vi "MiniCanSat 2018 V1.1.vi"() -> ()   [LabVIEW 2015]
uses:
  <vilib>/Instr/_visa.llb/VISA Configure Serial Port (Instr).vi
panel:
  out "Waveform Chart":dbl(graph)=145.63
  out "XY Graph":cluster{dbl[], dbl[]}(graph)={[100.91229833333334, 100.91229833333334, 100.91229999999999, 100.91229833333334, 100.912295, 100.912295, 100.912295, 100.912295, 100.912295, 100.91229666666668, 100.91229833333334, 100.91229833333334, 100.91229666666668, 100.91229833333334, 100.91229833333334, 100.91229999999999, 100.91229999999999, 100.91230166666668, 100.91230166666668, 100.91229999999999, 100.91229833333334, 100.912295, 100.91229333333334, 100.91229666666668, 100.91229666666668, 100.912295, 100.91229166666666, 100.91228833333335, 100.91228666666666, 100.91228500000001, 100.91228166666666, 100.91227833333332, 100.91227833333332, 100.91227666666667, 100.91227666666667, 100.91227500000001, 100.91227500000001, 100.91227333333333, 100.91227333333333, 100.91227333333333, 100.91227333333333, 100.91227333333333, 100.91227333333333, 100.91227333333333, 100.91227500000001, 100.91227500000001, 100.91227666666667, 100.91228166666666, 100.91228500000001, 100.91228833333335, 100.91229, 100.91229166666666, 100.91229166666666, 100.912295, 100.91229666666668, 100.91229999999999, 100.91230166666668, 100.91230166666668, 100.91229999999999, 100.91229833333334, 100.912295, 100.91229166666666, 100.91228666666666, 100.91228833333335, 100.91228666666666, 100.91228500000001, 100.91228166666666, 100.91227500000001, 100.91227500000001, 100.91227333333333, 100.91227666666667, 100.91227500000001, 100.91227333333333, 100.91227833333332, 100.91227500000001, 100.91227500000001, 100.91227833333332, 100.91228333333332, 100.91228666666666, 100.91229166666666, 100.912295, 100.91229833333334, 100.91230166666668, 100.91230333333333, 100.91230500000002, 100.91230666666667, 100.91230833333333, 100.91230833333333, 100.91231, 100.91231, 100.91231333333332, 100.912315, 100.91231333333332, 100.912315, 100.91231333333332, 100.91231333333332, 100.91231666666665, 100.91232166666666, 100.91232, 100.91232166666666, 100.91232166666666, 100.91232333333333, 100.91232333333333, 100.91232333333333, 100.91232666666669, 100.91233333333334, 100.91233333333334, 100.91233500000001, 100.91233666666668, 100.91233666666668, 100.91233500000001, 100.91233833333332, 100.91234166666666, 100.91234000000001, 100.91233833333332, 100.91234000000001, 100.91234166666666, 100.91234333333333, 100.91234333333333, 100.91234666666666, 100.91235, 100.91235166666665, 100.91235333333334, 100.91235333333334, 100.91235, 100.91234666666666, 100.912345, 100.91234000000001, 100.91233500000001, 100.91233333333334, 100.91233500000001, 100.91233333333334, 100.91233166666667, 100.91232999999998, 100.91232833333333, 100.91232666666669, 100.91233500000001, 100.91233166666667], [15.036158333333333, 15.036156666666667, 15.036156666666667, 15.036155, 15.036153333333335, 15.036155, 15.036155, 15.036155, 15.036155, 15.036155, 15.036155, 15.036155, 15.036153333333335, 15.036153333333335, 15.036153333333335, 15.036153333333335, 15.036153333333335, 15.036155, 15.036156666666667, 15.036158333333333, 15.036161666666665, 15.036161666666665, 15.03616333333333, 15.036166666666668, 15.036168333333334, 15.03617, 15.036173333333332, 15.036178333333332, 15.036181666666668, 15.036183333333334, 15.036183333333334, 15.036185, 15.036185, 15.036185, 15.036185, 15.036183333333334, 15.036183333333334, 15.036183333333334, 15.036181666666668, 15.036181666666668, 15.036180000000002, 15.036176666666666, 15.036174999999998, 15.036174999999998, 15.036176666666666, 15.036176666666666, 15.036178333333332, 15.036178333333332, 15.036178333333332, 15.036176666666666, 15.036174999999998, 15.036173333333332, 15.036171666666666, 15.03617, 15.036168333333334, 15.036166666666668, 15.036161666666665, 15.036156666666667, 15.036155, 15.036153333333335, 15.036153333333335, 15.036153333333335, 15.036151666666667, 15.036151666666667, 15.036153333333335, 15.036153333333335, 15.036155, 15.036156666666667, 15.036159999999999, 15.036159999999999, 15.03616333333333, 15.036165000000002, 15.036166666666668, 15.03617, 15.03617, 15.036171666666666, 15.036176666666666, 15.036181666666668, 15.036185, 15.036188333333333, 15.03619, 15.036193333333332, 15.036196666666667, 15.036198333333335, 15.036200000000001, 15.036203333333333, 15.036203333333333, 15.036204999999999, 15.036204999999999, 15.036204999999999, 15.036204999999999, 15.036203333333333, 15.036201666666667, 15.036201666666667, 15.036203333333333, 15.036204999999999, 15.036206666666665, 15.036210000000002, 15.036213333333334, 15.036218333333332, 15.036221666666666, 15.036221666666666, 15.036223333333332, 15.036223333333332, 15.036223333333332, 15.036223333333332, 15.036221666666666, 15.036219999999998, 15.036218333333332, 15.036216666666666, 15.036215, 15.036211666666668, 15.036210000000002, 15.036210000000002, 15.036206666666665, 15.036204999999999, 15.036204999999999, 15.036203333333333, 15.036203333333333, 15.036203333333333, 15.036204999999999, 15.036203333333333, 15.036203333333333, 15.036204999999999, 15.036204999999999, 15.036203333333333, 15.036203333333333, 15.036201666666667, 15.036201666666667, 15.036201666666667, 15.036201666666667, 15.036201666666667, 15.036201666666667, 15.036198333333335, 15.036195000000001, 15.036193333333332, 15.03619, 15.03619]}
  in  "file path":path=path "C:/Data"
  out "Height":dbl=145.63
  out "Longitude":string="100.91233167"
  out "Latitude":string="15.03619000"
  in  "stop":bool
  in  "VISA resource name":refnum<visa-resource-name>="COM6"
  # "Ground Station : Mini CANSAT 2018"
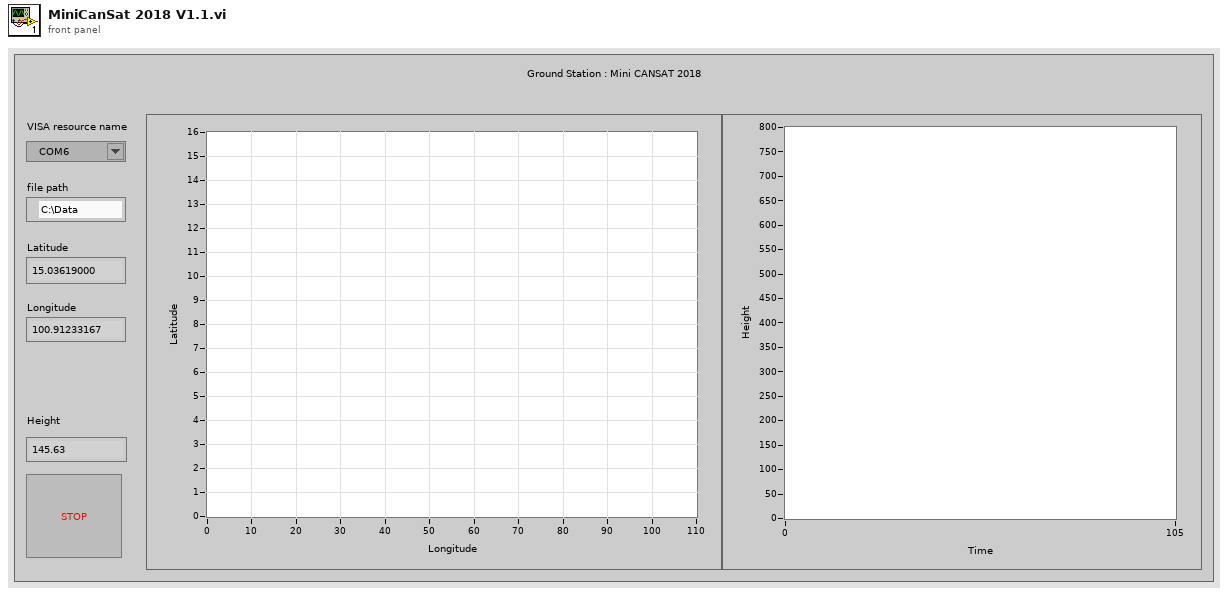
[diagram p1: front panel]
types:
  T1 = enum16{"open", "replace", "create", "open or create", "replace or create", "replace or create with confirmation"}
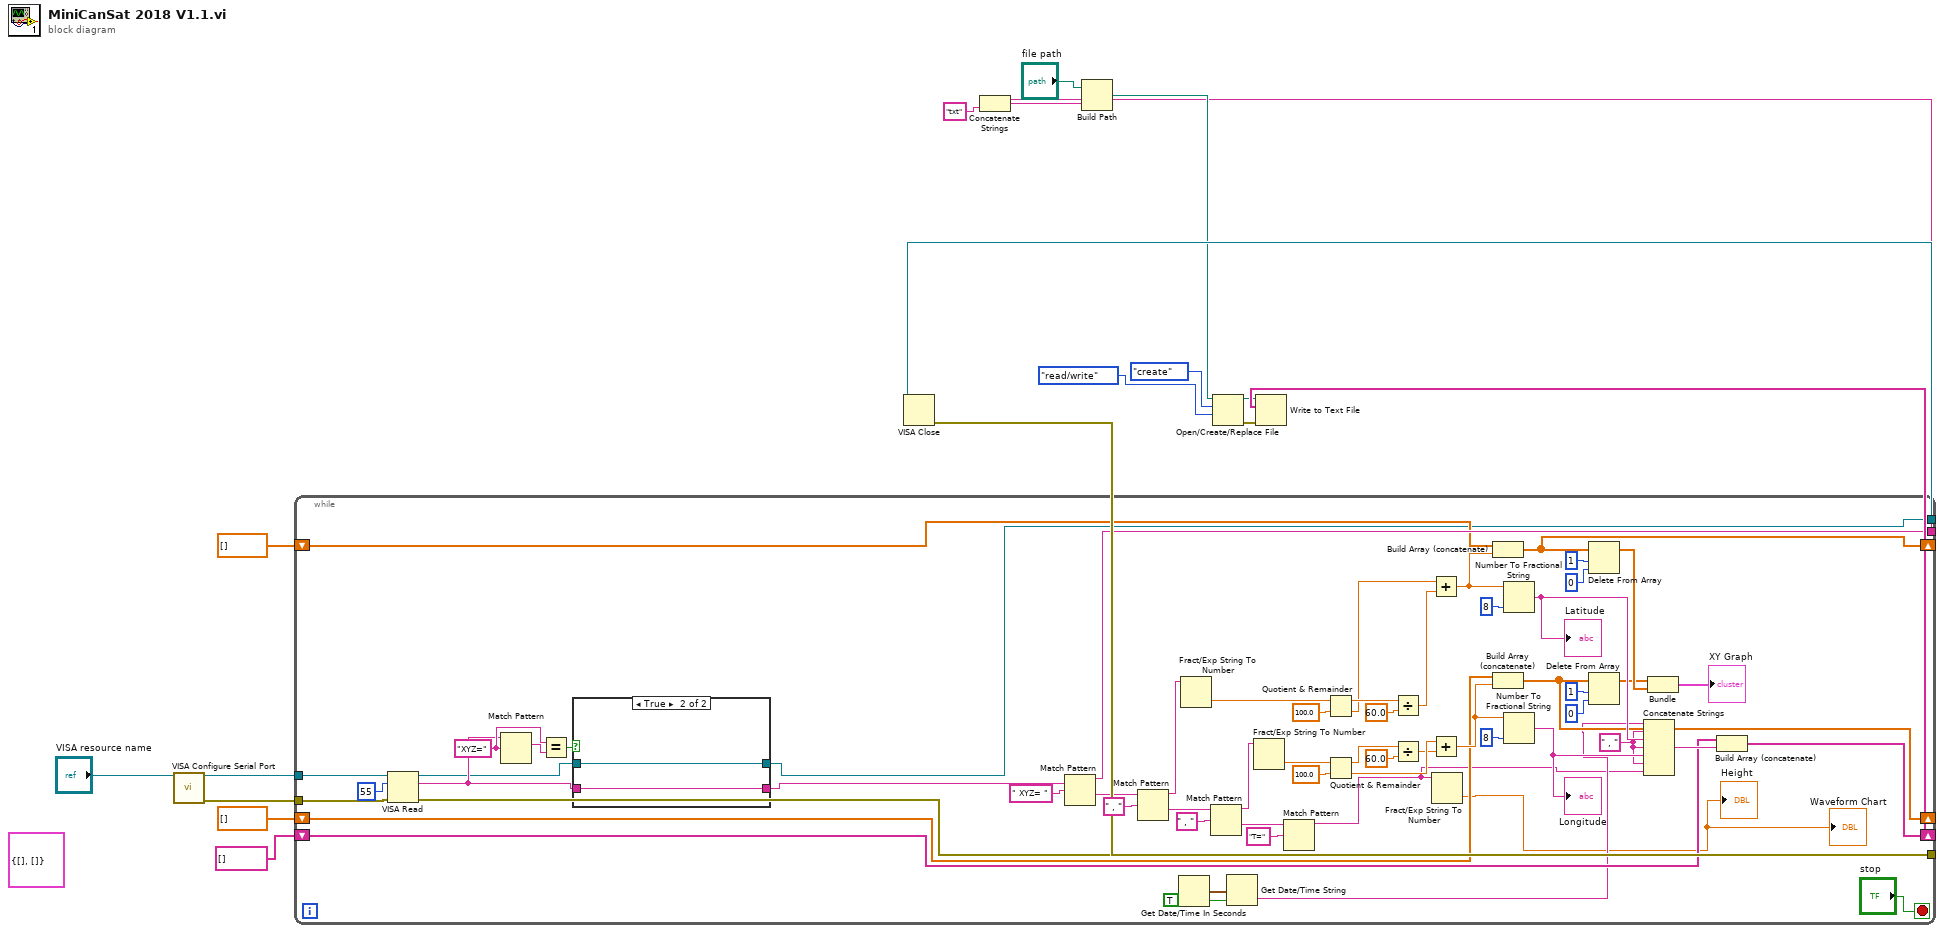
[diagram p0: block diagram]
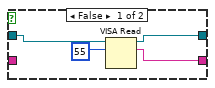
[diagram p2: hidden frame]
diagram:
  (unwired) cluster{dbl[], dbl[]} {[], []} ("XY Graph")
  n1 = call-poly "VISA Configure Serial Port"("VISA resource name"="VISA resource name") -> ("VISA resource name out"=w17:refnum<visa-resource-name>, "error out"=w16:errorcluster)  [unwired: 13 in]
  n2 = while {
    tunnel: w17 -> [w78]
    tunnel: w16 -> [w77]
    tunnel: [w22] -> w15
    tunnel: [w20] -> w14
    shift-right: [w48] -> w12
    shift-left: string[] [] -> [w49]
    tunnel: [w47] -> w5
    shift-right: [w36] -> _
    shift-left: dbl[] [] -> [w45]
    shift-right: [w41] -> _
    shift-left: dbl[] [] -> [w43]
    stop <- "stop" stop-if-true
    w26 = "XYZ=" ("regular expression")
    w30 = " , " ("string")
    n3 = VISA Read(VISA resource name=w78, byte count=u32 55, error in (no error)=w77) -> (VISA resource name out=w23:refnum<visa-resource-name>, read buffer=w25:string, error out=w20:errorcluster)  [unwired: 1 out]
    n4 = Match Pattern(string=w25, regular expression=w26) -> (match substring=w27:string)  [unwired: 1 in, 3 out]
    n5 = Equal?(x=w26, y=w27) -> (x = y?=w28:bool)
    n6 = case shown="True" w28 {
      tunnel: w25 -> [_ w84]
      tunnel: [w79 w84] -> w24
      tunnel: w23 -> [w81 w83]
      tunnel: [w80 w83] -> w22
      frame False {
        n7 = VISA Read(VISA resource name=w81, byte count=u32 55) -> (VISA resource name out=w80:refnum<visa-resource-name>, read buffer=w79:string)  [unwired: 1 in, 2 out]
      }
      frame True {
      }
    }
    n8 = Match Pattern(string=w24, regular expression=" XYZ= ") -> (before substring=w47:string, after substring=w73:string)  [unwired: 1 in, 2 out]
    n9 = Match Pattern(string=w73, regular expression=" , ") -> (before substring=w68:string, after substring=w70:string)  [unwired: 1 in, 2 out]
    n10 = Get Date/Time In Seconds() -> (seconds since 1Jan1904=w33:timestamp)
    n11 = Fract/Exp String To Number(string=w68) -> (number=w66:dbl)  [unwired: 3 in, 1 out]
    n12 = Match Pattern(string=w70, regular expression=" , ") -> (before substring=w67:string, after substring=w69:string)  [unwired: 1 in, 2 out]
    n13 = Get Date/Time String(seconds (now)=w33, want seconds? (F)=TRUE) -> (time string=w32:string)  [unwired: 1 in, 1 out]
    n14 = Fract/Exp String To Number(string=w67) -> (number=w63:dbl)  [unwired: 3 in, 1 out]
    n15 = Match Pattern(string=w69, regular expression="T=") -> (before substring=w29:string)  [unwired: 1 in, 3 out]
    n16 = Quotient & Remainder(x=w66, y=100.0) -> (x-y*floor(x/y)=w59:dbl, floor(x/y)=w55:dbl)
    n17 = Quotient & Remainder(x=w63, y=100.0) -> (x-y*floor(x/y)=w57:dbl, floor(x/y)=w54:dbl)
    n18 = Divide(x=w59, y=60.0) -> (x/y=w56:dbl)
    n19 = Divide(x=w57, y=60.0) -> (x/y=w53:dbl)
    n20 = Add(x=w55, y=w56) -> (x+y=w44:dbl)
    n21 = Add(x=w54, y=w53) -> (x+y=w46:dbl)
    n22 = Fract/Exp String To Number(string=w29) -> (number=→"Height" →"Waveform Chart":dbl)  [unwired: 3 in, 1 out]
    n23 = Build Array (concatenate)(w43, w44) -> (w41:dbl[])
    n24 = Build Array (concatenate)(w45, w46) -> (w36:dbl[])
    n25 = Number To Fractional String(number=w44, precision (6)=i16 8) -> (F-format string=w52:string)  [unwired: 2 in]
    "Latitude" <- w52
    n26 = Number To Fractional String(number=w46, precision (6)=i16 8) -> (F-format string=w51:string)  [unwired: 2 in]
    "Longitude" <- w51
    n27 = Delete From Array(array=w41, length=1, index=0) -> (array with subset deleted=w35:dbl[])  [unwired: 1 out]
    n28 = Delete From Array(array=w36, length=1, index=0) -> (array with subset deleted=w34:dbl[])  [unwired: 1 out]
    n29 = Concatenate Strings(w32, w30, w52, w30, w51, w30, w29) -> (w50:string)
    n30 = Bundle(w34, w35) -> (→"XY Graph":cluster{dbl[], dbl[]})  [unwired: 1 in]
    n31 = Build Array (concatenate)(w49, w50) -> (w48:string[])
  }
  n32 = VISA Close(VISA resource name=w15, error in (no error)=w14) -> ()  [unwired: 1 out]
  n33 = Concatenate Strings(w5, "txt" ("string")) -> (w4:string)
  n34 = Build Path(base path="file path", name or relative path=w4) -> (appended path=w7:path)
  n35 = Open/Create/Replace File(file path (use dialog)=w7, operation (0:open)=T1."create", access (0:read/write)=enum16{"read/write", "read-only", "write-only"}."read/write") -> (refnum out=w11:refnum<file>, error out=w10:errorcluster)  [unwired: 3 in, 1 out]
  n36 = Write to Text File(file (use dialog)=w11, text=w12, error in=w10) -> ()  [unwired: 1 in, 3 out]
